vi "FwdKin.vi"(8 "q2":dbl, 9 "q1":dbl, 11 "L":dbl) -> (0 "states vec":T1, 2 "theta":dbl, 3 "r":dbl)   [LabVIEW 2019]
uses:
  <vilib>/Analysis/Matrix/Datatypes/RealMatrix.ctl
  <vilib>/Analysis/Matrix/NI_Matrix.lvlib
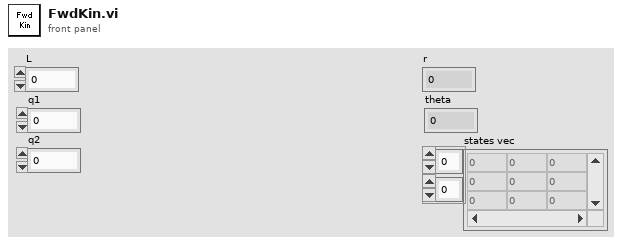
[diagram p1: front panel]
types:
  T1 = typedef "NI_Matrix.lvlib/RealMatrix.ctl" = dbl[][]
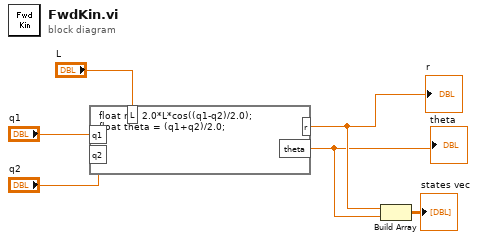
[diagram p0: block diagram]
diagram:
  n1 = formula code="float r = 2.0*L*cos((q1-q2)/2.0);\nfloat theta = (q1+q2)/2.0;"("q2"="q2", "L"="L", "q1"="q1") -> ("r"=w3:dbl, "theta"=w2:dbl)
  "r" <- w3
  "theta" <- w2
  n2 = Build Array(w3, w2) -> (→"states vec":T1)
